vi "MGI Read Key (Double[][]).vi"(7 "Section":string, 8 "error in (no error)":errorcluster, 9 "Default Value[][]":dbl[][](array[numeric]), 10 "Key":string, 11 "Refnum":T1) -> (0 "error out":errorcluster, 1 "Value[][]":dbl[][](array[numeric]) format="%.2f", 2 "Found?":bool, 3 "Refnum":T1)   [LabVIEW 2020]
doc: "Read a 2D float array key (actually a section) written by the matching Write VI.\n\nAuthored by David A. Moore\nsupport@mooregoodideas.com\nwww.mooregoodideas.com\n\nCopyright (c) 2010, Moore Good Ideas, Inc.\n\nAll rights reserved.\n\nRedistribution and use in source and binary forms, with or without modification, are permitted provided that the following conditions are met:\n\n * Redistributions of source code must retain the above copyright notice, this list of conditions and the following disclaimer.\n * Redistributions in binary form must reproduce the above copyright notice, this list of conditions and the following disclaimer in the documentation and/or other materials provided with the distribution.\n * Neither the name of Moore Good Ideas, Inc. nor the names of its contributors may be used to endorse or promote products derived from this software without specific prior written permission.\n\nTHIS SOFTWARE IS PROVIDED BY THE COPYRIGHT HOLDERS AND CONTRIBUTORS \"AS IS\" AND ANY EXPRESS OR IMPLIED WARRANTIES, INCLUDING, BUT NOT LIMITED TO, THE IMPLIED WARRANTIES OF MERCHANTABILITY AND FITNESS FOR A PARTICULAR PURPOSE ARE DISCLAIMED. IN NO EVENT SHALL THE COPYRIGHT OWNER OR CONTRIBUTORS BE LIABLE FOR ANY DIRECT, INDIRECT, INCIDENTAL, SPECIAL, EXEMPLARY, OR CONSEQUENTIAL DAMAGES (INCLUDING, BUT NOT LIMITED TO, PROCUREMENT OF SUBSTITUTE GOODS OR SERVICES; LOSS OF USE, DATA, OR PROFITS; OR BUSINESS INTERRUPTION) HOWEVER CAUSED AND ON ANY THEORY OF LIABILITY, WHETHER IN CONTRACT, STRICT LIABILITY, OR TORT (INCLUDING NEGLIGENCE OR OTHERWISE) ARISING IN ANY WAY OUT OF THE USE OF THIS SOFTWARE, EVEN IF ADVISED OF THE POSSIBILITY OF SUCH DAMAGE."
uses:
  <vilib>/Utility/config.llb/Config Data RefNum.ctl
  <vilib>/Utility/config.llb/Read Key (I32).vi
  <vilib>/Utility/config.llb/Read Key (Double).vi
  <vilib>/Utility/config.llb/NI_LVConfig.lvlib
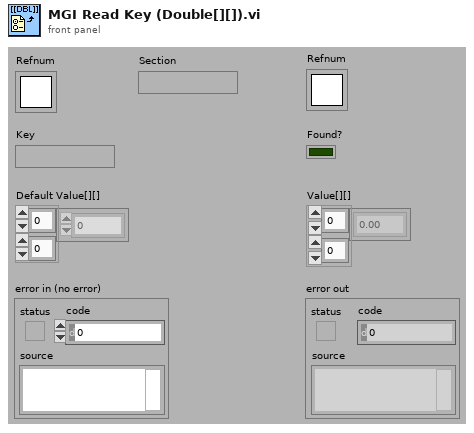
[diagram p1: front panel]
types:
  T1 = typedef "NI_LVConfig.lvlib/Config Data RefNum.ctl" = refnum<k1>
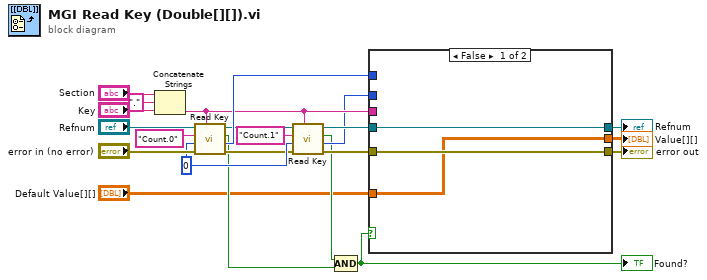
[diagram p0: block diagram]
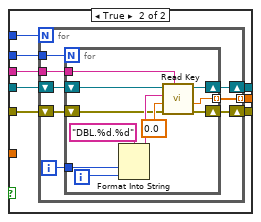
[diagram p2: hidden frame]
diagram:
  w14 = 0
  n1 = Concatenate Strings("Section", "." ("Substring"), "Key") -> (w9:string)
  n2 = call-poly <vilib>:"Read Key.vi"("section"=w9, "error in (no error)"="error in (no error)", "default value"=w14, "key"="Count.0", "refnum"="Refnum") -> ("error out"=w11:errorcluster, "value"=w13:i32, "found?"=w3:bool, "refnum out"=w10:T1)  [unwired: 3 in]
  n3 = call-poly <vilib>:"Read Key.vi"("section"=w9, "error in (no error)"=w11, "default value"=w14, "key"="Count.1", "refnum"=w10) -> ("error out"=w7:errorcluster, "value"=w5:i32, "found?"=w4:bool, "refnum out"=w8:T1)  [unwired: 3 in]
  n4 = Compound Arithmetic op=AND(w4, w3) -> (w2:bool)
  "Found?" <- w2
  n5 = case shown="False" w2 {
    tunnel: [w24 w33] -> w21
    tunnel: [w25 w32] -> w20
    tunnel: w13 -> [_ w31]
    tunnel: [w23 w30] -> w12
    tunnel: w9 -> [_ w29]
    tunnel: w8 -> [w25 w28]
    tunnel: w7 -> [w24 w27]
    tunnel: w5 -> [_ w26]
    tunnel: "Default Value[][]" -> [w23 _]
    frame False {
    }
    frame True {
      n6 = for {
        N: w31 -> [_]
        shift-right: [w35] -> w33
        shift-left: w27 -> [w37]
        shift-right: [w34] -> w32
        shift-left: w28 -> [w38]
        tunnel: w29 -> [w41]
        tunnel: [w39] -> w30 mode=indexing
        tunnel: w26 -> [w36]
        i -> [w40]
        n7 = for {
          N: w36 -> [_]
          tunnel: w41 -> [w52]
          tunnel: w40 -> [w51]
          tunnel: [w47] -> w39 mode=indexing
          shift-right: [w43] -> w35
          shift-left: w37 -> [w45]
          shift-right: [w42] -> w34
          shift-left: w38 -> [w44]
          i -> [w46]
          n8 = Format Into String(format string="DBL.%d.%d" ("Format String"), w51, w46) -> (resulting string=w50:string)  [unwired: 2 in, 1 out]
          n9 = call-poly <vilib>:"Read Key.vi"("section"=w52, "error in (no error)"=w45, "default value"=0.0, "key"=w50, "refnum"=w44) -> ("error out"=w43:errorcluster, "value"=w47:dbl, "refnum out"=w42:T1)  [unwired: 3 in, 1 out]
        }
      }
    }
  }
  "Value[][]" <- w12
  "error out" <- w21
  "Refnum" <- w20
